vi "Initialize UI.vi"(8 "error in (no error)":errorcluster, 11 "Application Data in":T1) -> (0 "error out":errorcluster, 3 "Application Data out":T1)   [LabVIEW 2017, in "DSF Mini Explorer.lvlib"]
uses:
  DSF Mini Explorer.lvlib
  Application Data.ctl
  VeriStand/Data Sharing Custom Device/Source/DSF Core.lvlibp/Classes/Configuration/Configuration Session.lvclass
  View Mode.ctl
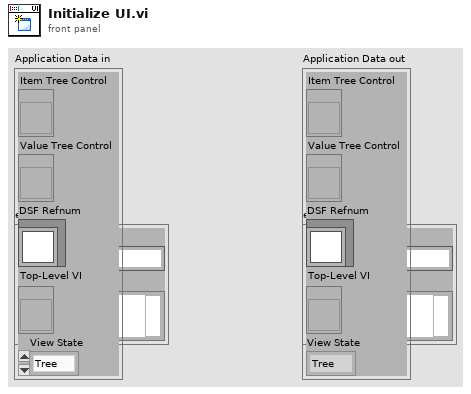
[diagram p1: front panel]
types:
  T1 = typedef "DSF Mini Explorer.lvlib/Application Data.ctl" = cluster{"Item Tree Control":refnum<vi>, "Value Tree Control":refnum<vi>, "DSF Refnum":refnum<class "Configuration Session.lvclass">, "Top-Level VI":refnum<vi>, "View State":T2}
  T2 = typedef "DSF Mini Explorer.lvlib/View Mode.ctl" = enum16{"Tree", "List"}
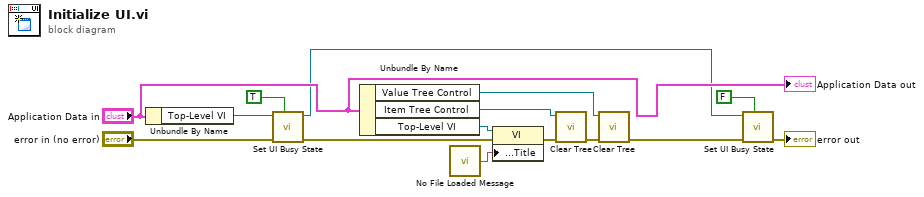
[diagram p0: block diagram]
diagram:
  n1 = Unbundle By Name("Application Data in") -> ("Top-Level VI"=w10:refnum<vi>)
  n2 = call "Set UI Busy State.vi"("Defer Panel Updates"=TRUE, "error in (no error)"="error in (no error)", "VI in"=w10) -> ("error out"=w13:errorcluster, "VI out"=w7:refnum<vi>)  [unwired: 7 in]
  n3 = Unbundle By Name("Application Data in") -> ("Value Tree Control"=w1:refnum<vi>, "Item Tree Control"=w6:refnum<vi>, "Top-Level VI"=w4:refnum<vi>)
  n4 = call "No File Loaded Message.vi"() -> ("no file loaded string"=w3:string)  [unwired: 1 in]
  n5 = property class="VI"(reference=w4, error in=w13, "Front Panel.Title"=w3) -> (error out=w5:errorcluster)  [unwired: 1 out]
  n6 = call "Clear Tree.vi"("error in (no error)"=w5, "TreeControl in"=w6) -> ("error out"=w2:errorcluster)  [unwired: 9 in]
  n7 = call "Clear Tree.vi"("error in (no error)"=w2, "TreeControl in"=w1) -> ("error out"=w14:errorcluster)  [unwired: 9 in]
  n8 = call "Set UI Busy State.vi"("Defer Panel Updates"=FALSE, "error in (no error)"=w14, "VI in"=w7) -> ("error out"=→"error out":errorcluster)  [unwired: 7 in, 1 out]
  "Application Data out" <- "Application Data in"
